vi "Main.vi"() -> ()   [LabVIEW 2017]
panel:
  out "sortie d'erreur":errorcluster
  out "tableau d'octets non signés 2":u8[](array[numeric]) format="%x"
  in  "Error In":errorcluster caption="entrée d'erreur (pas d'erreur)"
  in  "Port":u16=3000
  in  "TCP Address":string="192.168.1.4"
  in  "Cluster":T1
  out "chaîne 2":string
  out "octets écrits":i32
  in  "Bouton Stop":bool
  # "SainSmart iMatic RJ45 TCP/IP Remote Control Board for 16-Ch Relay"
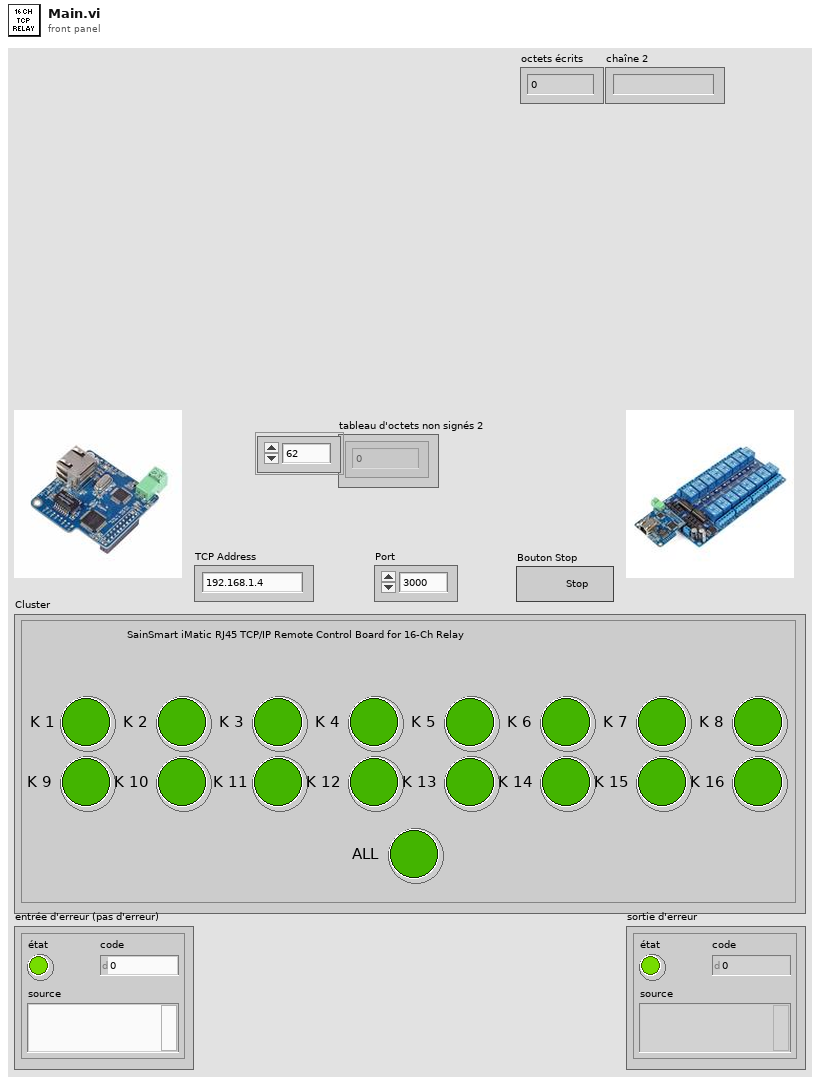
[diagram p1: front panel]
types:
  T1 = cluster{"K 1":bool, "K 2":bool, "K 3":bool, "K 4":bool, "K 5":bool, "K 6":bool, "K 7":bool, "K 8":bool, "K 9":bool, "K 10":bool, "K 11":bool, "K 12":bool, "K 13":bool, "K 14":bool, "K 15":bool, "K 16":bool, "ALL":bool}
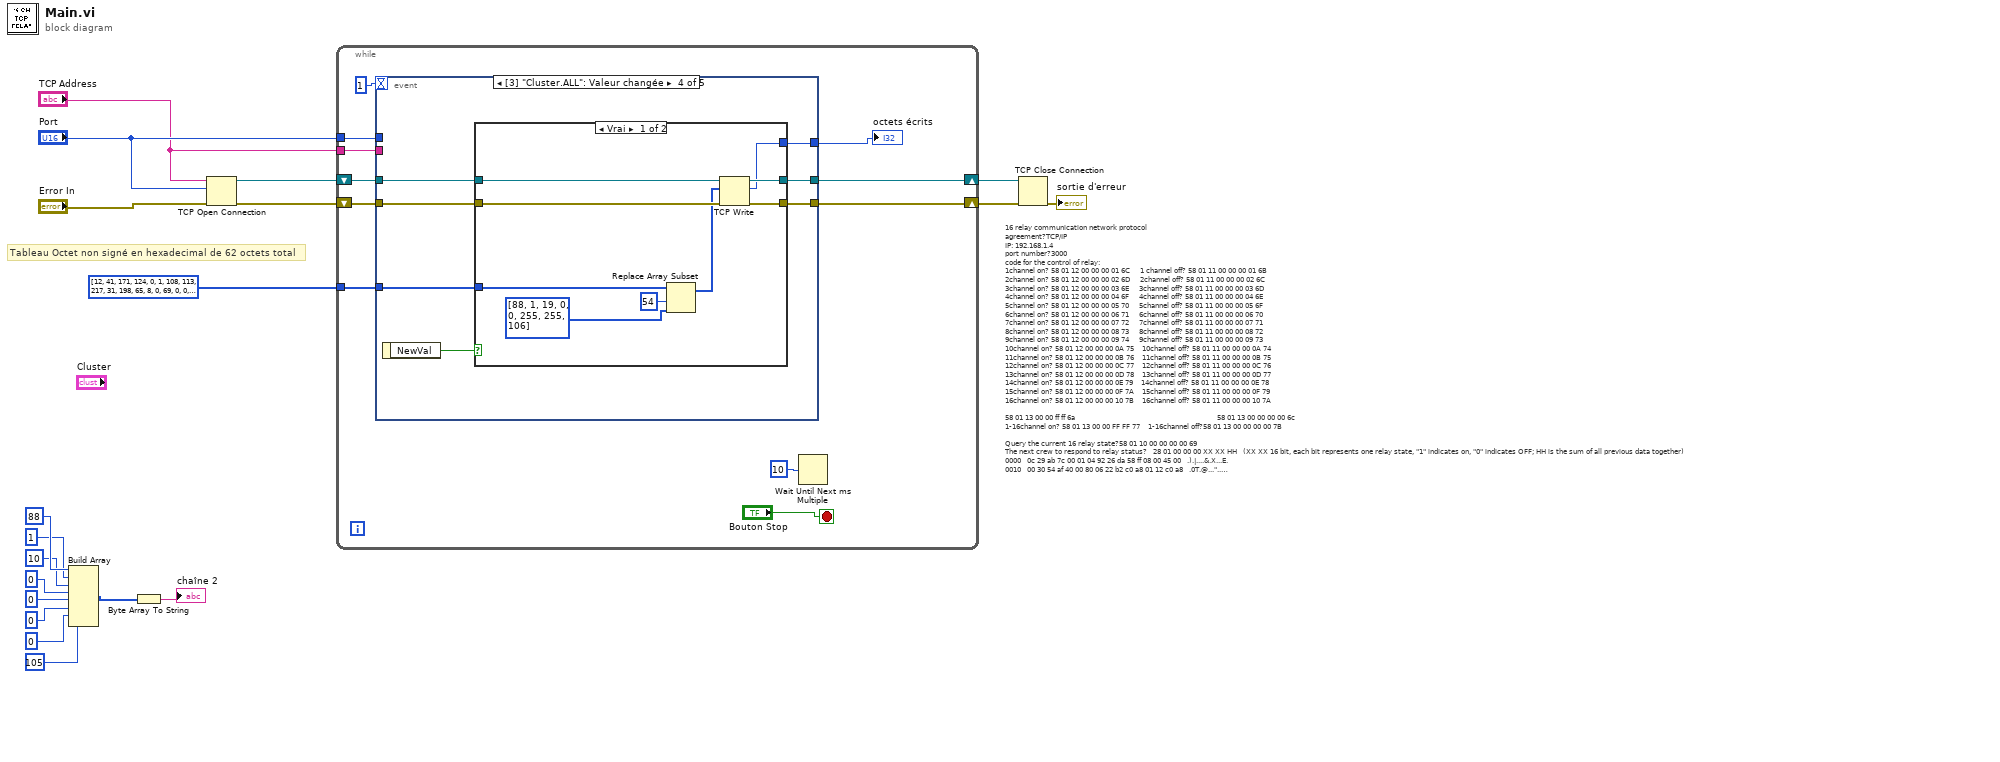
[diagram p0: block diagram]
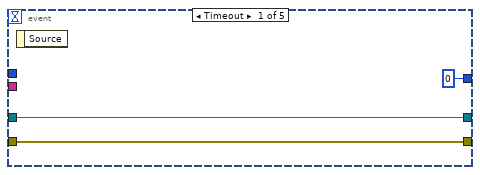
[diagram p2: hidden frame]
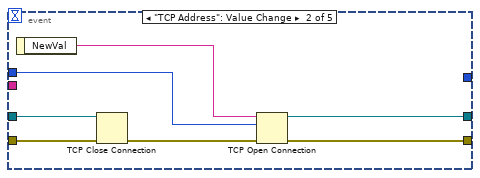
[diagram p3: hidden frame]
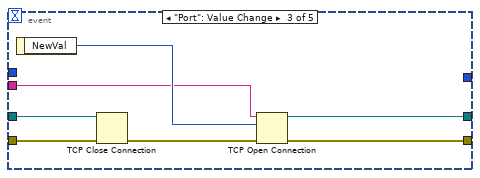
[diagram p4: hidden frame]
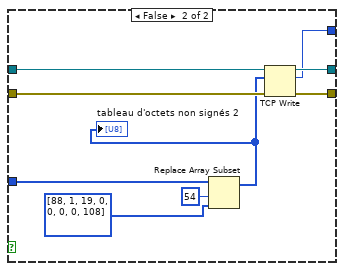
[diagram p5: hidden frame]
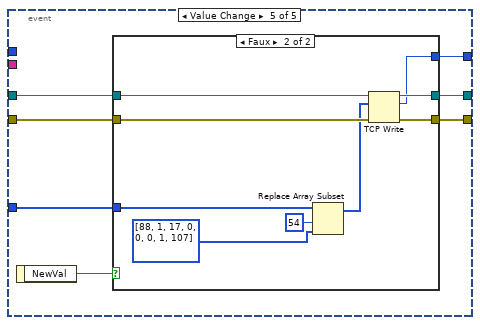
[diagram p6: hidden frame]
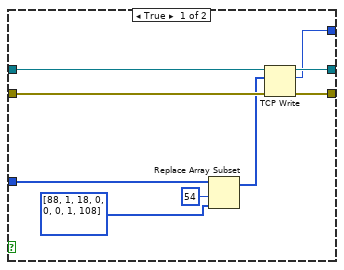
[diagram p7: hidden frame]
diagram:
  # "16 relay communication network protocol\nagreement?TCP/IP\nIP: 192.168.1.4\nport number?3000 \ncode for the control of relay:\n1channel on? 58 01 12 00 00 00 01 6C     1 channel off? 58 01 11 00 00 00 01 6B\n2channel on? 58 01 12 00 00 00 02 6D     2channel off? 58 01 11 00 00 00 02 6C\n3channel on? 58 01 12 00 00 00 03 6E     3channel off? 58 01 11 00 00 00 03 6D\n4channel on? 58 01 12 00 00 00 04 6F     4channel off? 58 01 11 00 00 00 04 6E\n5channel on? 58 01 12 00 00 00 05 70     5channel off? 58 01 11 00 00 00 05 6F\n6channel on? 58 01 12 00 00 00 06 71     6channel off? 58 01 11 00 00 00 06 70\n7channel on? 58 01 12 00 00 00 07 72     7channel off? 58 01 11 00 00 00 07 71\n8channel on? 58 01 12 00 00 00 08 73     8channel off? 58 01 11 00 00 00 08 72\n9channel on? 58 01 12 00 00 00 09 74     9channel off? 58 01 11 00 00 00 09 73\n10channel on? 58 01 12 00 00 00 0A 75    10channel off? 58 01 11 00 00 00 0A 74\n11channel on? 58 01 12 00 00 00 0B 76    11channel off? 58 01 11 00 00 00 0B 75\n12channel on? 58 01 12 00 00 00 0C 77    12channel off? 58 01 11 00 00 00 0C 76\n13channel on? 58 01 12 00 00 00 0D 78    13channel off? 58 01 11 00 00 00 0D 77\n14channel on? 58 01 12 00 00 00 0E 79    14channel off? 58 01 11 00 00 00 0E 78\n15channel on? 58 01 12 00 00 00 0F 7A    15channel off? 58 01 11 00 00 00 0F 79\n16channel on? 58 01 12 00 00 00 10 7B    16channel off? 58 01 11 00 00 00 10 7A\n\n58 01 13 00 00 ff ff 6a                                                                       58 01 13 00 00 00 00 6c\n1-16channel on? 58 01 13 00 00 FF FF 77    1-16channel off?58 01 13 00 00 00 00 7B\n\nQuery the current 16 relay state?58 01 10 00 00 00 00 69\nThe next crew to respond to relay status?   28 01 00 00 00 XX XX HH   (XX XX 16 bit, each bit represents one relay state, \"1\" indicates on, \"0\" indicates OFF; HH is the sum of all previous data together)\n0000   0c 29 ab 7c 00 01 04 92 26 da 58 ff 08 00 45 00   .).|....&.X...E.\n0010   00 30 54 af 40 00 80 06 22 b2 c0 a8 01 12 c0 a8   .0T.@...\".......\n0020   01 04 8c f1 0b b8 80 16 0d 85 e7 86 8e a2 50 18   ..............P.\n0030   fa d8 29 ab 00 00 58 01 13 00 00 ff ff 6a         ..)...X......j\n0000   0c 29 ab 7c 00 01 04 92 26 da 58 ff 08 00 45 00   .).|....&.X...E.\n0010   00 30 54 b1 40 00 80 06 22 b0 c0 a8 01 12 c0 a8   .0T.@...\".......\n0020   01 04 8c f1 0b b8 80 16 0d 8d e7 86 8e aa 50 18   ..............P.\n0030   fa d0 29 a1 00 00 58 01 13 00 00 00 00 6c         ..)...X......l"
  # "Tableau Octet non signé en hexadecimal de 62 octets total"
  n1 = Build Array(u8 88 ("élément"), u8 1 ("élément"), u8 10 ("élément"), u8 0 ("élément"), u8 0 ("élément"), u8 0 ("élément"), u8 0 ("élément"), u8 105 ("élément")) -> (w1:u8[])
  n2 = Byte Array To String(unsigned byte array=w1) -> (string=→"chaîne 2":string)
  n3 = TCP Open Connection(address="TCP Address", remote port or service name="Port", error in (no error)="Error In") -> (connection ID=w17:refnum<k5>, error out=w16:errorcluster)  [unwired: 2 in]
  n4 = while {
    shift-right: [w24] -> w19
    shift-left: w17 -> [w27]
    shift-right: [w23] -> w18
    shift-left: w16 -> [w26]
    tunnel: "Port" -> [w25]
    tunnel: "TCP Address" -> [w22]
    tunnel: u8[] [12, 41, 171, 124, 0, 1, 108, 113, 217, 31, 198, 65, 8, 0, 69, 0, 0, 48, 111, 152, 64, 0, 128, 6, 7, 193, 192, 168, 1, 26, 192, 168, 1, 4, 214, 0, 11, 184, 114, 220, 20, 37, 193, 253, 187, 189, 80, 24, 250, 216, 223, 153, 0, 0, 88, 1, 19, 0, 0, 0, 0, 108] ("tableau d'octets non signés 2") -> [w21]
    stop <- "Bouton Stop" stop-if-true
    n5 = event shown="[3] \"Cluster.ALL\": Valeur changée" {
      selector: _ -> [_ _ _ _ _]
      dyn-events: _ -> [_ _ _ _ _]
      timeout: 1 -> [_ _ _ _ _]
      tunnel: w27 -> [w33 w40 w47 w50 w75]
      tunnel: w26 -> [w32 w39 w46 w49 w74]
      tunnel: w25 -> [_ w37 _ _ _]
      tunnel: [w33 w35 w44 w52 w77] -> w24
      tunnel: [w32 w34 w43 w51 w76] -> w23
      tunnel: w22 -> [_ _ w41 _ _]
      tunnel: w21 -> [_ _ _ w53 w78]
      tunnel: [0 ("bytes written") _ _ w48 w73] -> w20
      event Timeout {
        n6 = event-data() -> ()  [unwired: 1 in, 1 out]
      }
      event "TCP Address": Value Change {
        n7 = event-data() -> ("NewVal"=w38:string)  [unwired: 1 in]
        n8 = TCP Close Connection(connection ID=w40, error in (no error)=w39) -> (error out=w36:errorcluster)  [unwired: 1 in, 1 out]
        n9 = TCP Open Connection(address=w38, remote port or service name=w37, error in (no error)=w36) -> (connection ID=w35:refnum<k5>, error out=w34:errorcluster)  [unwired: 2 in]
      }
      event "Port": Value Change {
        n10 = event-data() -> ("NewVal"=w42:u16)  [unwired: 1 in]
        n11 = TCP Close Connection(connection ID=w47, error in (no error)=w46) -> (error out=w45:errorcluster)  [unwired: 1 in, 1 out]
        n12 = TCP Open Connection(address=w41, remote port or service name=w42, error in (no error)=w45) -> (connection ID=w44:refnum<k5>, error out=w43:errorcluster)  [unwired: 2 in]
      }
      event "Cluster.ALL": Value Change {
        n13 = event-data() -> ("NewVal"=w54:bool)  [unwired: 1 in]
        n14 = case shown="Vrai" w54 {
          tunnel: w53 -> [w63 w72]
          tunnel: [w62 w71] -> w52
          tunnel: [w61 w70] -> w51
          tunnel: w50 -> [w60 w69]
          tunnel: w49 -> [w59 w68]
          tunnel: [w57 w66] -> w48
          frame True {
            n15 = Replace Array Subset(array=w63, new element=u8[] [88, 1, 19, 0, 0, 255, 255, 106] ("tableau ajouté"), index=54 ("indice")) -> (w56:u8[])
            n16 = TCP Write(connection ID=w60, data in=w56, error in (no error)=w59) -> (connection ID out=w62:refnum<k5>, bytes written=w57:i32, error out=w61:errorcluster)  [unwired: 1 in]
          }
          frame False {
            n17 = Replace Array Subset(array=w72, new element=u8[] [88, 1, 19, 0, 0, 0, 0, 108] ("tableau ajouté"), index=54 ("indice")) -> (w64:u8[])
            "tableau d'octets non signés 2" <- w64
            n18 = TCP Write(connection ID=w69, data in=w64, error in (no error)=w68) -> (connection ID out=w71:refnum<k5>, bytes written=w66:i32, error out=w70:errorcluster)  [unwired: 1 in]
          }
        }
      }
      event "Cluster.K 1": Value Change {
        n19 = event-data() -> ("NewVal"=w79:bool)  [unwired: 1 in]
        n20 = case shown="Faux" w79 {
          tunnel: w78 -> [w88 w97]
          tunnel: [w87 w96] -> w77
          tunnel: [w86 w95] -> w76
          tunnel: w75 -> [w85 w94]
          tunnel: w74 -> [w84 w93]
          tunnel: [w82 w91] -> w73
          frame True {
            n21 = Replace Array Subset(array=w88, new element=u8[] [88, 1, 18, 0, 0, 0, 1, 108] ("tableau ajouté"), index=54 ("indice")) -> (w81:u8[])
            n22 = TCP Write(connection ID=w85, data in=w81, error in (no error)=w84) -> (connection ID out=w87:refnum<k5>, bytes written=w82:i32, error out=w86:errorcluster)  [unwired: 1 in]
          }
          frame False {
            n23 = Replace Array Subset(array=w97, new element=u8[] [88, 1, 17, 0, 0, 0, 1, 107] ("tableau ajouté"), index=54 ("indice")) -> (w90:u8[])
            n24 = TCP Write(connection ID=w94, data in=w90, error in (no error)=w93) -> (connection ID out=w96:refnum<k5>, bytes written=w91:i32, error out=w95:errorcluster)  [unwired: 1 in]
          }
        }
      }
    }
    "octets écrits" <- w20
    n25 = Wait Until Next ms Multiple(millisecond multiple=u32 10 ("n millisecondes")) -> ()  [unwired: 1 out]
  }
  n26 = TCP Close Connection(connection ID=w19, error in (no error)=w18) -> (error out=→"sortie d'erreur":errorcluster)  [unwired: 1 in, 1 out]
